vi "RT Control Loop.vi"(8 "error in (no error)":errorcluster, 10 "FIFO Buffers":refnum<k33>[](array[refnum]), 11 "Queue in":refnum<queue>) -> ()   [LabVIEW 2014]
uses:
  RT Stop.vi
  RT Tags.vi
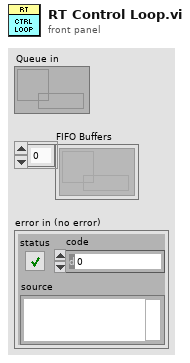
[diagram p1: front panel]
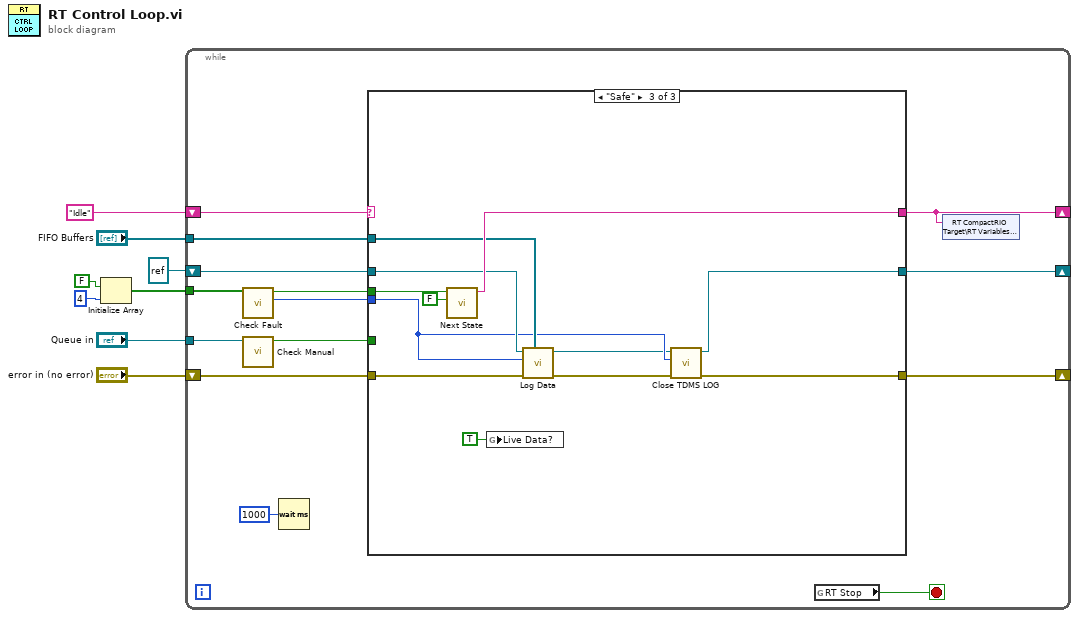
[diagram p0: block diagram]
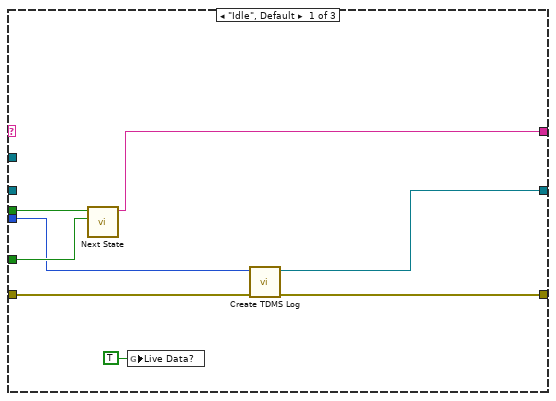
[diagram p2: hidden frame]
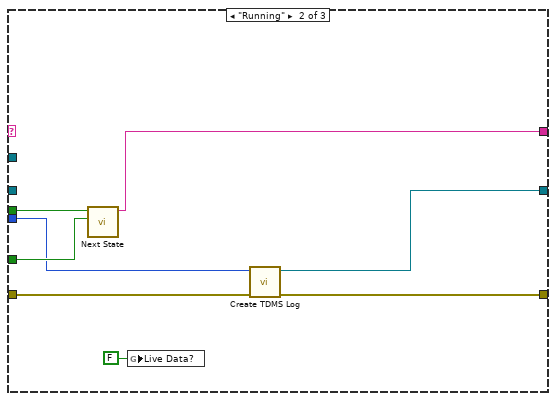
[diagram p3: hidden frame]
diagram:
  n1 = Initialize Array(FALSE, 4 ("dimension size")) -> (w5:bool[])
  n2 = while {
    shift-right: [w12] -> _
    shift-left: "Idle" -> [w21]
    tunnel: "FIFO Buffers" -> [w20]
    tunnel: w5 -> [w19]
    tunnel: "Queue in" -> [w15]
    shift-right: [w13] -> _
    shift-left: "error in (no error)" -> [w14]
    shift-right: [w11] -> _
    shift-left: refnum<k34> refnum ("Refnum out") -> [w10]
    stop <- w22 stop-if-true
    n3 = call "Check Fault.vi"("Array"=w19) -> ("Fault Index"=w17:i32, "Fault?"=w18:bool)  [unwired: 9 in]
    n4 = call "Check Manual.vi"("Queue in"=w15) -> ("Manual"=w16:bool)  [unwired: 10 in]
    n5 = Wait (ms)(milliseconds to wait=u32 1000) -> ()  [unwired: 1 out]
    n6 = case shown="\"Safe\"" w21 {
      tunnel: w20 -> [_ _ w46]
      tunnel: w18 -> [w30 w38 w50]
      tunnel: w17 -> [w24 w32 w41]
      tunnel: w16 -> [w29 w37 _]
      tunnel: [w28 w36 w49] -> w12
      tunnel: w14 -> [w26 w34 w44]
      tunnel: [w25 w33 w42] -> w13
      tunnel: [w23 w31 w39] -> w11
      tunnel: w10 -> [_ _ w45]
      frame "Idle", Default {
        n7 = call "Next State.vi"("Manual"=w29, "Fault?"=w30) -> ("String"=w28:string)  [unwired: 9 in]
        n8 = global write "RT Tags.vi" "Live Data?"(TRUE ("Live Data?")) -> ()
        n9 = call "Create TDMS Log.vi"("error in (no error)"=w26, "Fault Index"=w24) -> ("error out"=w25:errorcluster, "Refnum out"=w23:refnum<k34>)  [unwired: 8 in]
      }
      frame "Running" {
        n10 = call "Next State.vi"("Manual"=w37, "Fault?"=w38) -> ("String"=w36:string)  [unwired: 9 in]
        n11 = global write "RT Tags.vi" "Live Data?"(FALSE ("Live Data?")) -> ()
        n12 = call "Create TDMS Log.vi"("error in (no error)"=w34, "Fault Index"=w32) -> ("error out"=w33:errorcluster, "Refnum out"=w31:refnum<k34>)  [unwired: 8 in]
      }
      frame "Safe" {
        n13 = call "Next State.vi"("Manual"=FALSE, "Fault?"=w50) -> ("String"=w49:string)  [unwired: 9 in]
        n14 = global write "RT Tags.vi" "Live Data?"(TRUE ("Live Data?")) -> ()
        n15 = call "Log Data.vi"("FIFO Buffers"=w46, "error in (no error)"=w44, "Fault Index"=w41, "Refnum in"=w45) -> ("error out"=w43:errorcluster, "Refnum out"=w40:refnum<k34>)  [unwired: 6 in]
        n16 = call "Close TDMS LOG.vi"("error in (no error)"=w43, "Fault Index"=w41, "Refnum in"=w40) -> ("error out"=w42:errorcluster, "Refnum out"=w39:refnum<k34>)  [unwired: 7 in]
      }
    }
    n17 = global read "RT Stop.vi" "RT Stop"() -> (w22:bool)
    n18 = shared-variable "RT CompactRIO Target\\RT Variables.lvlib\\Status"(w12) -> ()  [unwired: 1 in, 1 out]
  }
